vi "误差分析.vi"(11 "Array输入":refnum<vi>) -> (2 "平均值":dbl, 3 "A类不确定度":dbl)   [LabVIEW 2016]
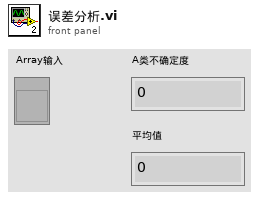
[diagram p1: front panel]
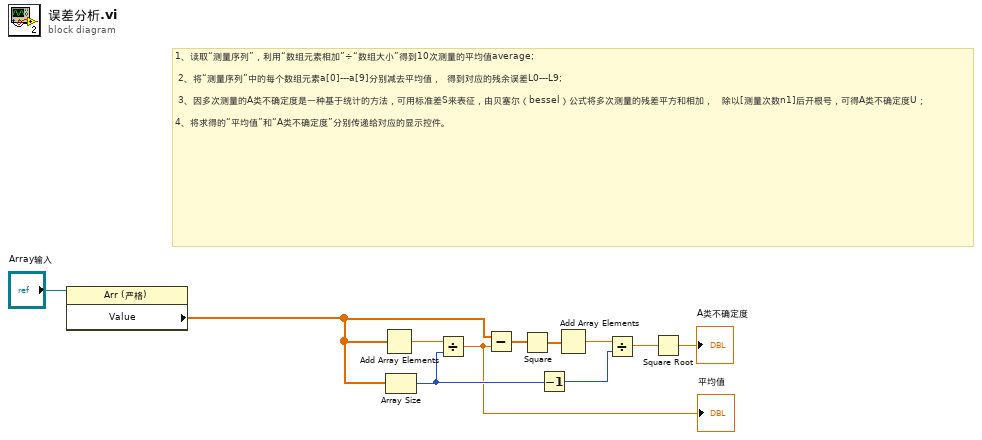
[diagram p0: block diagram]
diagram:
  # "1、读取“测量序列”，利用“数组元素相加”÷“数组大小”得到10次测量的平均值average;\n\n 2、将“测量序列”中的每个数组元素a[0]---a[9]分别减去平均值，  得到对应的残余误差L0---L9;\n\n 3、因多次测量的A类不确定度是一种基于统计的方法，可用标准差S来表征，由贝塞尔（bessel）公式将多次测量的残差平方和相加，   除以[测量次数n1]后开根号，可得A类不确定度U；\n\n4、将求得的“平均值”和“A类不确定度”分别传递给对应的显示控件。"
  n1 = property class="Arr (严格)"(reference="Array输入") -> ("Value"=w1:dbl[])  [unwired: 1 in, 2 out]
  n2 = Add Array Elements(numeric array=w1) -> (sum=w3:dbl)
  n3 = Array Size(array=w1) -> (size(s)=w10:i32)
  n4 = Divide(x=w3, y=w10) -> (x/y=w4:dbl)
  "平均值" <- w4
  n5 = Subtract(x=w1, y=w4) -> (x-y=w7:dbl[])
  n6 = Square(x=w7) -> (x^2=w8:dbl[])
  n7 = Decrement(x=w10) -> (x-1=w11:i32)
  n8 = Add Array Elements(numeric array=w8) -> (sum=w9:dbl)
  n9 = Divide(x=w9, y=w11) -> (x/y=w5:dbl)
  n10 = Square Root(x=w5) -> (sqrt(x)=→"A类不确定度":dbl)
